vi "Close.vi"(8 "error in (no error)":errorcluster, 11 "ENET in":refnum<class "ENET_BS120x.lvclass">) -> (0 "error out":errorcluster, 3 "ENET out":refnum<class "ENET_BS120x.lvclass">)   [LabVIEW 2021, in "BS120x Driver.lvlib" / "ENET_BS120x.lvclass"]
uses:
  ENET_BS120x.lvclass
  ENET_BS120x.lvclass/ENET_BS120x.ctl
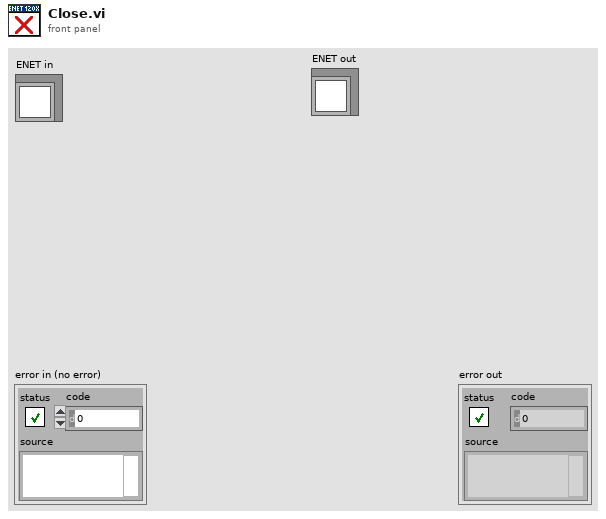
[diagram p1: front panel]
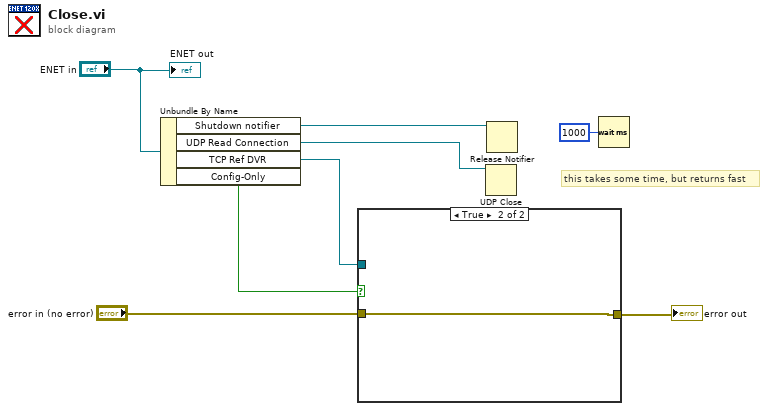
[diagram p0: block diagram]
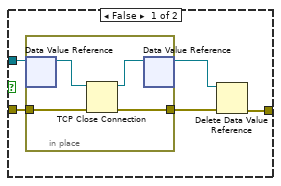
[diagram p2: hidden frame]
diagram:
  # "this takes some time, but returns fast"
  n1 = Unbundle By Name("ENET in") -> ("Shutdown notifier"=w8:refnum<notifier>, "UDP Read Connection"=w7:refnum<k16>, "TCP Ref DVR"=w4:refnum<data-value>, "Config-Only"=w1:bool)
  n2 = case shown="True" w1 {
    tunnel: w4 -> [w13 _]
    tunnel: "error in (no error)" -> [w12 w18]
    tunnel: [w11 w18] -> w2
    frame False {
      n3 = in-place {
        in-place-border: w12 -> [w17]
        in-place-border: [w14] -> w10
        n4 = in-place-dvr #1(w13) -> (w16:refnum<k5>)  [unwired: 1 out]
        n5 = TCP Close Connection(connection ID=w16, error in (no error)=w17) -> (connection ID out=w15:refnum<k5>, error out=w14:errorcluster)  [unwired: 1 in]
        n6 = in-place-dvr #1(w15) -> (w9:refnum<data-value>)  [unwired: 1 out]
      }
      n7 = Delete Data Value Reference(data value reference=w9, error in=w10) -> (error out=w11:errorcluster)  [unwired: 1 out]
    }
    frame True {
    }
  }
  "error out" <- w2
  n8 = UDP Close(connection ID=w7) -> ()  [unwired: 1 in, 2 out]
  n9 = Release Notifier(notifier=w8) -> ()  [unwired: 2 in, 3 out]
  n10 = Wait (ms)(milliseconds to wait=u32 1000) -> ()  [unwired: 1 out]
  "ENET out" <- "ENET in"
